vi "tablogin_2009.vi"() -> ()   [LabVIEW 2011]
panel:
  in  "Tab Control":enum32{"Login", "Main"}(tab)
  in  "login":bool
  in  "Password":string
  in  "Username":string
  out "Numeric":dbl
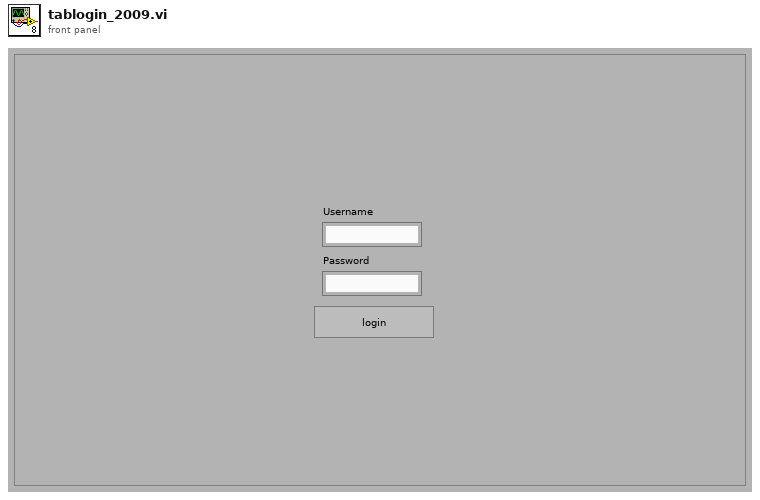
[diagram p1: front panel]
types:
  T1 = typedef "LVRemotePanelConnectionsTypeDef.ctl" = cluster{"VI Name":string, "Remote":string, "UserName":string, "Port":i32, "Status":enum32{"Viewing", "Waiting For Control", "Controlling"}, "Create Time":timestamp, "Status Time":timestamp, "Control End Time":timestamp}[]
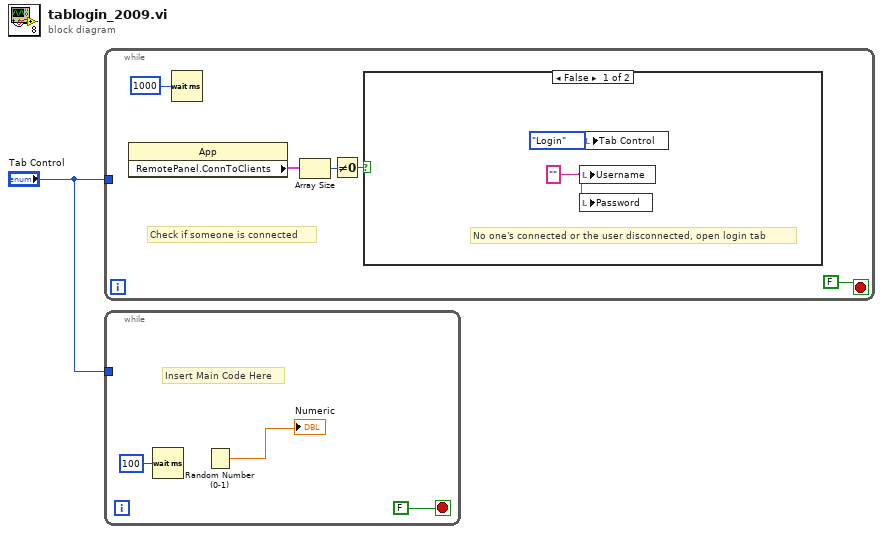
[diagram p0: block diagram]
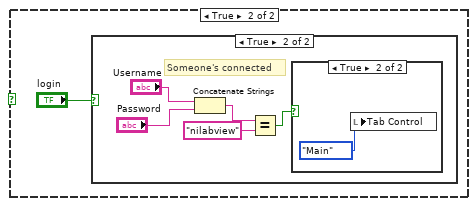
[diagram p2: hidden frame]
diagram:
  n1 = while {
    tunnel: "Tab Control" -> [_]
    stop <- FALSE stop-if-true
    # "Check if someone is connected"
    n2 = property class="App"() -> ("RemotePanel.ConnToClients"=w5:T1)  [unwired: 2 in, 2 out]
    n3 = Wait (ms)(milliseconds to wait=u32 1000) -> ()  [unwired: 1 out]
    n4 = Array Size(array=w5) -> (size(s)=w4:i32)
    n5 = Not Equal To 0?(x=w4) -> (x != 0?=w3:bool)
    n6 = case shown="False" w3 {
      frame False {
        w8 = ""
        # "No one's connected or the user disconnected, open login tab"
        n7 = local write "Username"(w8) -> ()
        n8 = local write "Password"(w8) -> ()
        n9 = local write "Tab Control"(enum32{"Login", "Main"}."Login" ("Tab Control")) -> ()
      }
      frame True {
        # "Someone's connected"
        n10 = case shown="True" "login" {
          frame False {
          }
          frame True {
            n11 = Concatenate Strings("Username", "Password") -> (w12:string)
            n12 = Equal?(x=w12, y="nilabview") -> (x = y?=w10:bool)
            n13 = case shown="True" w10 {
              frame False {
              }
              frame True {
                n14 = local write "Tab Control"(enum32{"Login", "Main"}."Main" ("Tab Control")) -> ()
              }
            }
          }
        }
      }
    }
  }
  n15 = while {
    tunnel: "Tab Control" -> [_]
    stop <- FALSE stop-if-true
    # "Insert Main Code Here"
    n16 = Wait (ms)(milliseconds to wait=u32 100) -> ()  [unwired: 1 out]
    n17 = Random Number (0-1)() -> (number: 0 to 1=→"Numeric":dbl)
  }
